vi "Request to Message Data.vi"(8 "error in (no error)":errorcluster, 11 "JSON String":string) -> (0 "error out":errorcluster, 3 "msg data":variant)   [LabVIEW 2020]
uses:
  Lib/JSON-RPC/Classes/Request/Request.lvclass
  Lib/JSON-RPC/Classes/Request/Request.lvclass/Request.ctl
  Lib/JSON-RPC/Classes/params/params.To JSON Tree.vi
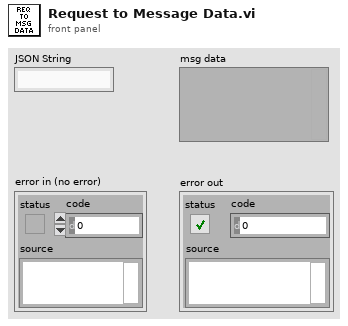
[diagram p1: front panel]
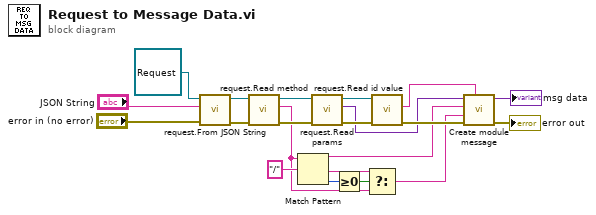
[diagram p0: block diagram]
diagram:
  n1 = call "request.From JSON String.vi"("error in (no error)"="error in (no error)", "JSON String"="JSON String", "Request in"=refnum<class "Request.lvclass"> refnum) -> ("error out"=w18:errorcluster, "Request out"=w17:refnum<class "Request.lvclass">)  [unwired: 7 in]
  n2 = call "request.Read method.vi"("error in (no error)"=w18, "Request in"=w17) -> ("error out"=w19:errorcluster, "method"=w3:string, "Request out"=w14:refnum<class "Request.lvclass">)  [unwired: 7 in]
  n3 = Match Pattern(string=w3, regular expression="/") -> (before substring=w4:string, after substring=w1:string, offset past match=w6:i32)  [unwired: 1 in, 1 out]
  n4 = call "request.Read params.vi"("error in (no error)"=w19, "Request in"=w14) -> ("error out"=w20:errorcluster, "params out"=w8:variant, "Request out"=w15:refnum<class "Request.lvclass">)  [unwired: 7 in]
  n5 = Greater Or Equal To 0?(x=w6) -> (x >= 0?=w5:bool)
  n6 = Select(t=w1, s=w5, f=w3) -> (s? t:f=w2:string)
  n7 = call "request.Read id value.vi"("error in (no error)"=w20, "Request in"=w15) -> ("error out"=w11:errorcluster, "value"=w9:string)  [unwired: 7 in, 1 out]
  n8 = call "Create module message.vi"("ID"=w9, "error in (no error)"=w11, "method"=w2, "module"=w4, "params"=w8) -> ("error out"=→"error out":errorcluster, "message data"=→"msg data":variant)  [unwired: 5 in]
